vi "_MobileTest_GetMappedPartitionID.vi"() -> (2 "ID":u32[](array[numeric]))   [LabVIEW 2019]
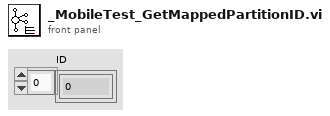
[diagram p1: front panel]
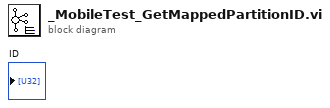
[diagram p0: block diagram]
diagram:
